vi "RSNRPZ Get Zeroing Complete State.vi"(8 "error in (no error)":errorcluster, 10 "Channel (1)":i32=1, 11 "VISA session":refnum<visa-resource-name> caption="VISA resource name") -> (0 "error out":errorcluster, 2 "Zeroing Complete":bool, 3 "dup VISA session":refnum<visa-resource-name> caption="VISA resource name")   [LabVIEW 2010]
doc: "This function should be used for polling whether a previously started zero calibration has already finished. Zero calibration is an asynchronous operation and may take some seconds until it completes. See the example code under RSNRPZ Zero.vi on how to conduct a sensor zeroing calibration."
uses:
  rsnrpz_32.dll
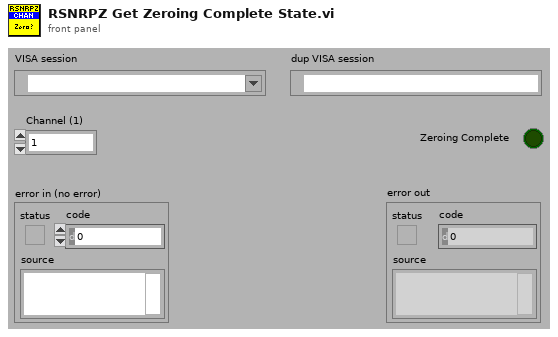
[diagram p1: front panel]
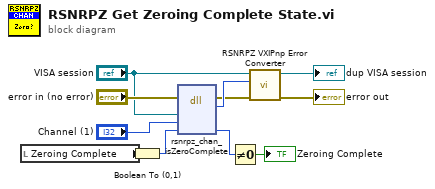
[diagram p0: block diagram]
diagram:
  n1 = local read "Zeroing Complete"() -> (w9:bool)
  n2 = Boolean To (0,1)(Boolean=w9) -> (0, 1=w6:i16)
  n3 = dll-call lib="rsnrpz_32.dll" fn="rsnrpz_chan_isZeroComplete"(error in="error in (no error)", "VISA Session"="VISA session", "Channel"="Channel (1)", "Zeroing Complete"=w6) -> (error out=w5:errorcluster, "Status"=w11:i32, "Zeroing Complete"=w8:u16)  [unwired: 4 in, 1 out]
  n4 = Not Equal To 0?(x=w8) -> (x != 0?=→"Zeroing Complete":bool)
  n5 = call <instrlib>:"RSNRPZ VXIPnp Error Converter.vi"("error in"=w5, "VXIPnp error code"=w11, "VISA session"="VISA session") -> ("error out"=→"error out":errorcluster, "dup VISA session"=→"dup VISA session":refnum<visa-resource-name>)  [unwired: 7 in]
